vi "Split Fit PPMS Hall.vi"(11 "Inut file path":path=path "\\\\myhome\\NHMFL/Projects/Pressure/Code/Alex/Hall_fitted_CeHx/Hallfit_cehx_feb24/Hall_CeHx_90p9K_Feb24.tdms") -> ()   [LabVIEW 2024]
panel:
  out "Output file path":path
  out "Temperature":cluster{dbl[], dbl[]}(graph) caption="XY Graph"
  in  "Temperature":string="T"
  out "Slope":dbl format="%#_6p"
  in  "Low field cut off":dbl=10.0
  out "Rxy(+B) - Rxy(-B)":cluster{"Binned data":dbl[], dbl[]}[](graph) caption="XY Graph"
  in  "Bin size":dbl=0.05
  in  "Save?":bool
  in  "Y":string="LakeShore 370 (18) R"
  in  "X":string="B"
  out "Split and binned +B and -B":cluster{dbl[], dbl[]}[](graph) caption="XY Graph"
  in  "group name in":string="p"
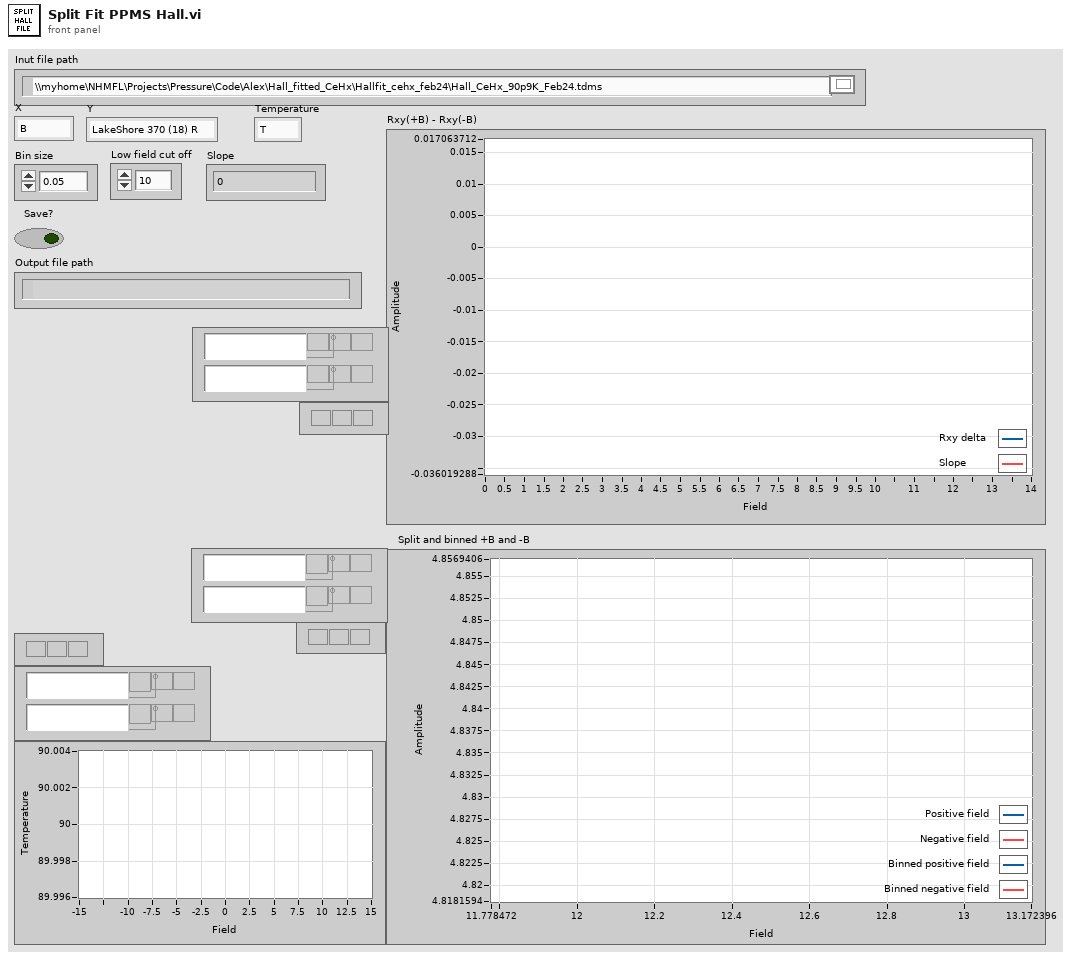
[diagram p1: front panel]
types:
  T1 = enum16{"open", "open or create", "create or replace", "create", "open (read-only)"}
  T2 = cluster{"Output low array":dbl[], "Output low array":dbl[]}
  T3 = cluster{"Output high array":dbl[], "Output high array":dbl[]}
  T4 = cluster{"Binned data":dbl[], "Binned data":dbl[]}
  T5 = cluster{"Binned data":dbl[], "Binned data":dbl[]}[]
  T6 = enum16{"open", "replace", "create", "open or create", "replace or create", "replace or create with confirmation"}
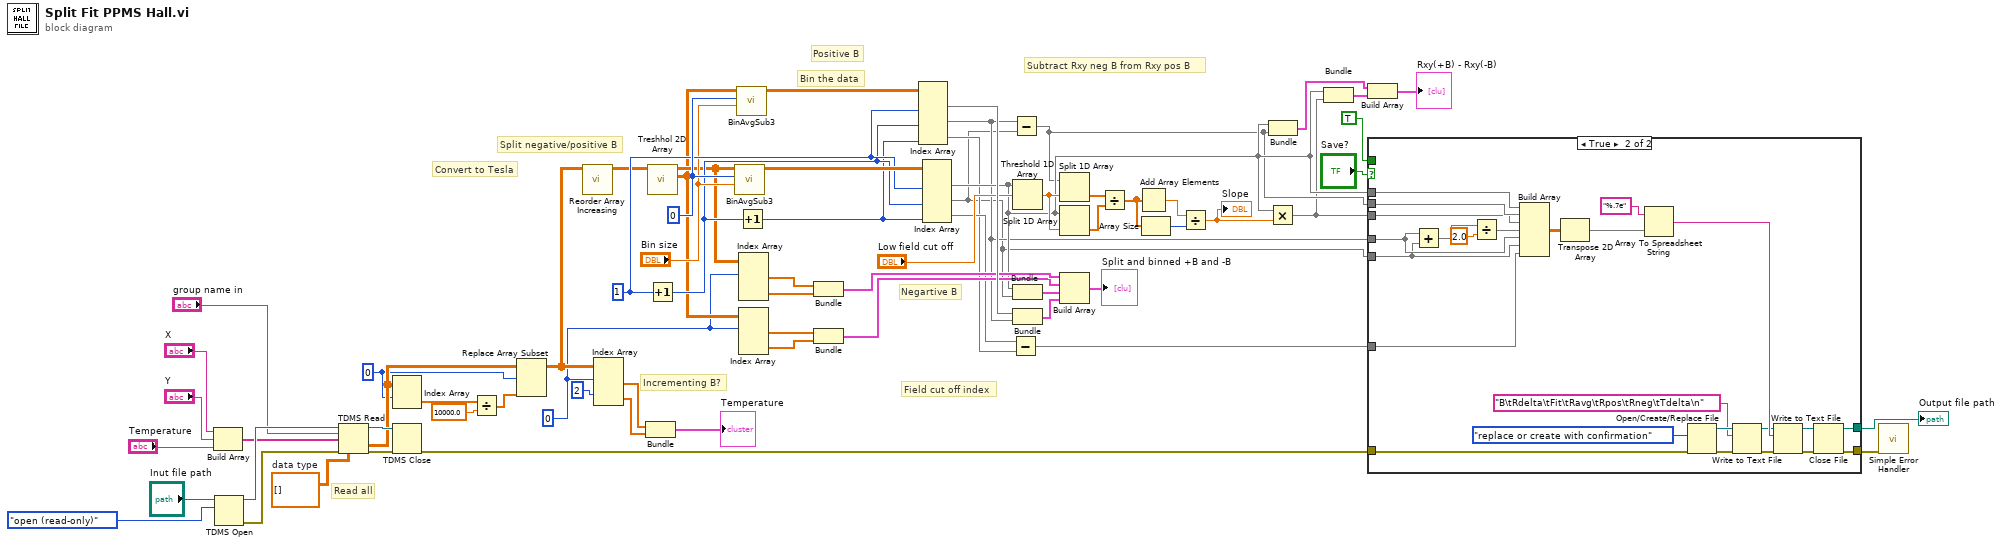
[diagram p0: block diagram]
diagram:
  w6 = 0 ("index (row)")
  w15 = 0 ("index (row)")
  w20 = dbl[][] []  # data type
  w59 = 1 ("disabled index (col)")
  w61 = 0 ("X coumn index")
  # "Positive B"
  # "Field cut off index"
  # "Subtract Rxy neg B from Rxy pos B"
  # "Negartive B"
  # "Bin the data"
  # "Split negative/positive B"
  # "Convert to Tesla"
  # "Incrementing B?"
  # "Read all"
  n1 = Build Array("X", "Y", "Temperature") -> (w22:string[])
  n2 = TDMS Open(10:T1."open (read-only)" ("operation (0:open)"), 11:"Inut file path") -> (0:w27:errorcluster, 3:w25:refnum<k34>)  [unwired: 5 in]
  n3 = TDMS Read(0:w25, 5:"group name in", 7:w22, 11:w27, 12:w20) -> (4:w24:refnum<k34>, 10:w16:dbl[][], 15:w26:errorcluster)  [unwired: 3 in, 3 out]
  n4 = Index Array(array=w16, index (row)=w15) -> (element=w17:dbl[])  [unwired: 1 in]
  n5 = TDMS Close(8:w26, 11:w24) -> (0:w43:errorcluster)  [unwired: 1 out]
  n6 = Divide(x=w17, y=10000.0) -> (x/y=w14:dbl[])
  n7 = Replace Array Subset(array=w16, new element=w14, index (row)=w15) -> (w7:dbl[][])  [unwired: 1 in]
  n8 = call "Reorder Array Increasing.vi"("Array"=w7) -> ("Output array"=w19:dbl[][])  [unwired: 10 in]
  n9 = Index Array(array=w7, index (row) #1=w6, index (row) #2=2 ("index (row)")) -> (element #1=w4:dbl[], element #2=w3:dbl[])  [unwired: 2 in]
  n10 = Bundle("data type"=w4, "data type"=w3) -> (→"Temperature":cluster{"data type":dbl[], "data type":dbl[]})  [unwired: 1 in]
  n11 = call "Treshhol 2D Array.vi"("Array"=w19) -> ("Output high array"=w10:dbl[][], "Output low array"=w13:dbl[][])  [unwired: 9 in]
  n12 = Increment(x=w59) -> (x+1=w35:i32)
  n13 = call "BinAvgSub3.vi"("Bin size"="Bin size", "X coumn index"=w61, "Data in"=w13) -> ("Binned data"=w62:dbl[][])  [unwired: 2 in, 6 out]
  n14 = call "BinAvgSub3.vi"("Bin size"="Bin size", "X coumn index"=w61, "Data in"=w10) -> ("Binned data"=w60:dbl[][])  [unwired: 2 in, 6 out]
  n15 = Increment(x=w35) -> (x+1=w34:i32)
  n16 = Index Array(array=w13, index (row) #1=w6) -> (element #1=w12:dbl[], element #2=w11:dbl[])  [unwired: 3 in]
  n17 = Index Array(array=w10, index (row) #1=w6) -> (element #1=w9:dbl[], element #2=w8:dbl[])  [unwired: 3 in]
  n18 = Bundle("Output low array"=w12, "Output low array"=w11) -> (w56:T2)  [unwired: 1 in]
  n19 = Bundle("Output high array"=w9, "Output high array"=w8) -> (w55:T3)  [unwired: 1 in]
  n20 = Index Array(array=w60, index (col) #1=w59, index (col) #2=w35, index (col) #3=w34) -> (element #1=w58:dbl[], element #2=w2:dbl[], element #3=w32:dbl[])  [unwired: 3 in]
  n21 = Index Array(array=w62, index (col) #1=w59, index (col) #2=w35, index (col) #3=w34) -> (element #1=w38:dbl[], element #2=w1:dbl[], element #3=w33:dbl[])  [unwired: 3 in]
  n22 = Subtract(x=w33, y=w32) -> (x-y=w31:dbl[])
  n23 = Subtract(x=w2, y=w1) -> (x-y=w37:dbl[])
  n24 = Threshold 1D Array(2:"Low field cut off", 3:w38) -> (0:w52:dbl)  [unwired: 1 in]
  n25 = Bundle("Binned data"=w38, "Binned data"=w1) -> (w65:T4)  [unwired: 1 in]
  n26 = Bundle("Binned data"=w58, "Binned data"=w2) -> (w63:T4)  [unwired: 1 in]
  n27 = Split 1D Array(array=w37, index=w52) -> (second subarray=w51:dbl[])  [unwired: 1 out]
  n28 = Split 1D Array(array=w38, index=w52) -> (second subarray=w50:dbl[])  [unwired: 1 out]
  n29 = Build Array(w56, w55, w65, w63) -> (→"Split and binned +B and -B":T5)
  n30 = Divide(x=w51, y=w50) -> (x/y=w49:dbl[])
  n31 = Add Array Elements(numeric array=w49) -> (sum=w48:dbl)
  n32 = Array Size(array=w49) -> (size(s)=w47:i32)
  n33 = Divide(x=w48, y=w47) -> (x/y=w46:dbl)
  "Slope" <- w46
  n34 = Multiply(x=w38, y=w46) -> (x*y=w36:dbl[])
  n35 = Bundle("Binned data"=w38, w37) -> (w54:cluster{"Binned data":dbl[], dbl[]})  [unwired: 1 in]
  n36 = Bundle("Binned data"=w38, w36) -> (w44:cluster{"Binned data":dbl[], dbl[]})  [unwired: 1 in]
  n37 = Build Array(w54, w44) -> (→"Rxy(+B) - Rxy(-B)":cluster{"Binned data":dbl[], dbl[]}[])
  n38 = case shown="True" "Save?" {
    tunnel: w43 -> [w68 w90]
    tunnel: [w68 w77] -> w41
    tunnel: TRUE ("append to file? (new file:F)") -> [_ _]
    tunnel: w38 -> [_ w92]
    tunnel: w37 -> [_ w91]
    tunnel: w36 -> [_ w88]
    tunnel: w2 -> [_ w73]
    tunnel: w1 -> [_ w72]
    tunnel: w31 -> [_ w87]
    tunnel: [_ w75] -> w30
    frame False {
    }
    frame True {
      n39 = Add(x=w73, y=w72) -> (x+y=w71:dbl[])
      n40 = Divide(x=w71, y=2.0 ("element")) -> (x/y=w69:dbl[])
      n41 = Build Array(w92, w91, w88, w69, w73, w72, w87) -> (w84:dbl[][])
      n42 = Transpose 2D Array(2D array=w84) -> (transposed array=w83:dbl[][])
      n43 = Array To Spreadsheet String(array=w83, 3:"%.7e" ("format (%.3f)")) -> (spreadsheet string=w80:string)  [unwired: 1 in]
      n44 = Open/Create/Replace File(error in=w90, operation (0:open)=T6."replace or create with confirmation") -> (refnum out=w89:refnum<file>, error out=w85:errorcluster)  [unwired: 4 in, 1 out]
      n45 = Write to Text File(file (use dialog)=w89, text="B\tRdelta\tFit\tRavg\tRpos\tRneg\tTdelta\n", error in=w85) -> (refnum out=w79:refnum<file>, error out=w81:errorcluster)  [unwired: 1 in, 1 out]
      n46 = Write to Text File(file (use dialog)=w79, text=w80, error in=w81) -> (refnum out=w76:refnum<file>, error out=w78:errorcluster)  [unwired: 1 in, 1 out]
      n47 = Close File(refnum=w76, error in=w78) -> (path=w75:path, error out=w77:errorcluster)
    }
  }
  "Output file path" <- w30
  n48 = call <vilib>:"Simple Error Handler.vi"("error in (no error)"=w41) -> ()  [unwired: 4 in, 5 out]
